vi "Read Unique Employees.vi"(8 "Error In":errorcluster, 11 "DVR In":refnum<data-value>) -> (0 "Error Out":errorcluster, 2 "Unique Employees":string[][](array[string]), 3 "DVR Out":refnum<data-value>)   [LabVIEW 2017, in "Data Operations.lvlib"]
uses:
  Data Operations.lvlib
  Private Controls/Report Data Cluster.ctl
  Private Controls/Data Raw.ctl
panel:
  out "Data":T1[](array[typedef])
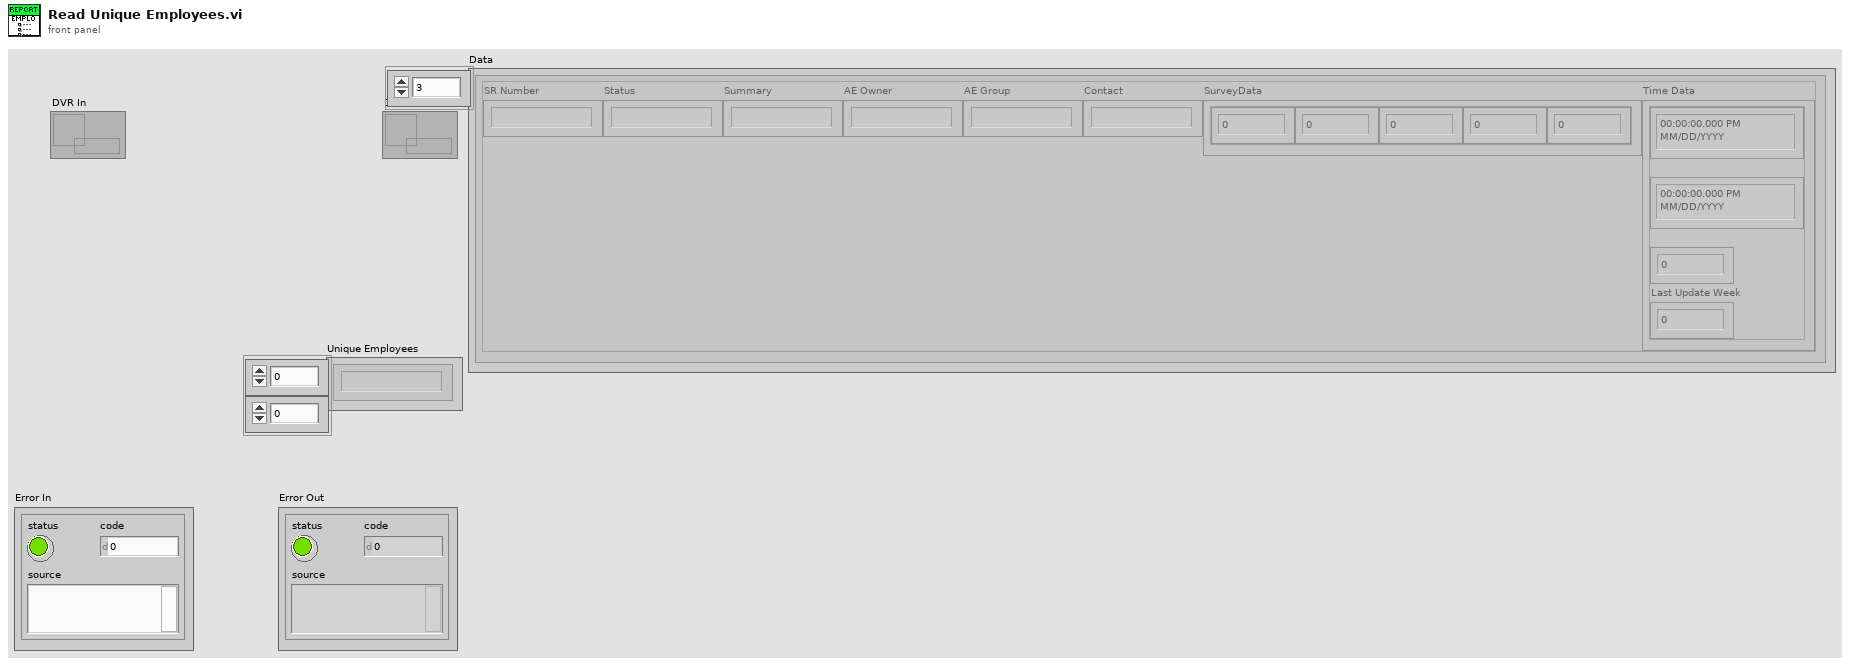
[diagram p1: front panel]
types:
  T1 = typedef "Data Operations.lvlib/Data Raw.ctl" = cluster{"SR Number":string, "Status":string, "Summary":string, "AE Owner":string, "AE Group":string, "Contact":string, "SurveyData":cluster{"Resolution Time":dbl, "Total Satisfaction":dbl, "Response Time":dbl, "Courtesy":dbl, "Problem Solved":dbl}, "Time Data":cluster{"Last Update Date":timestamp, "Creation Date":timestamp, "Creation week":u8, "Last Update Week":u8}}
  T2 = typedef "Data Operations.lvlib/Report Data Cluster.ctl" = cluster{"Headers":cluster{"Start Date":timestamp, "End Date":timestamp, "SR Status String":string[], "AE Owner String":string[]}, "Data":T1[]}
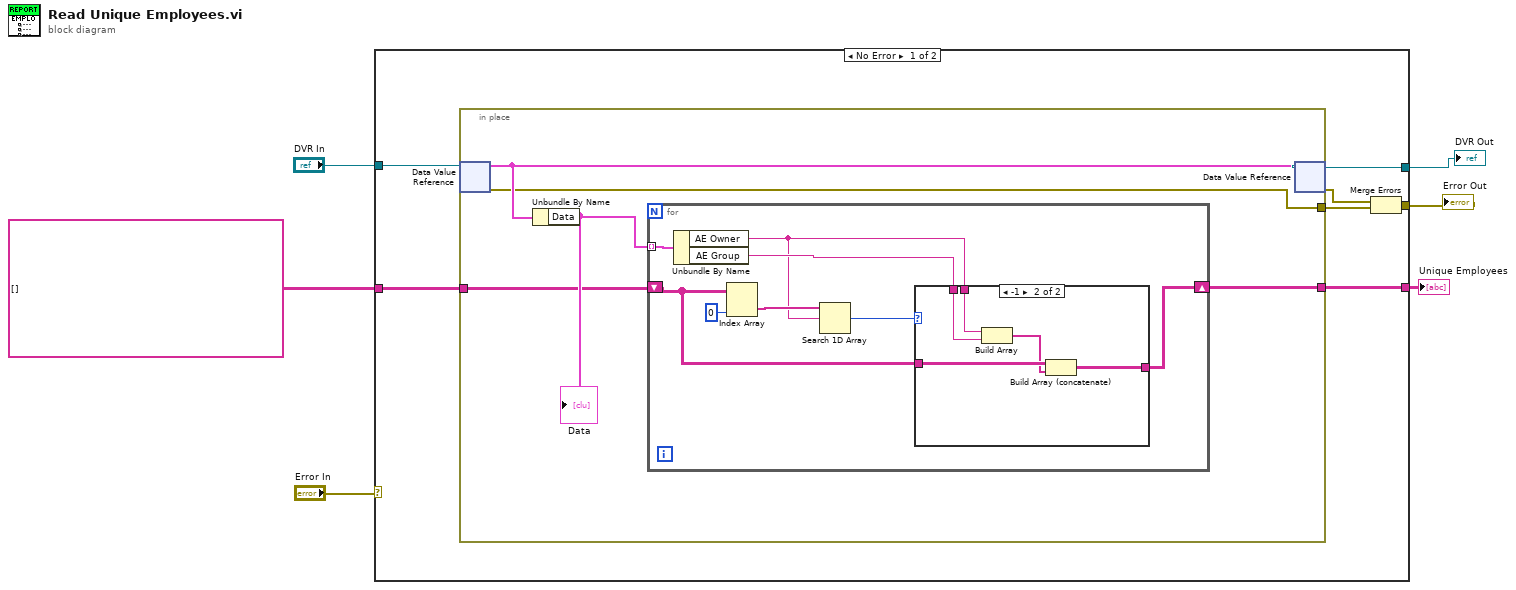
[diagram p0: block diagram]
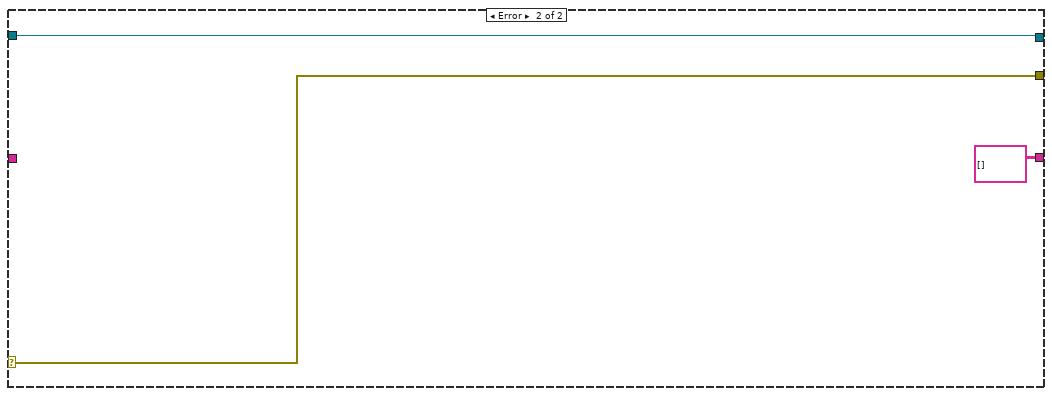
[diagram p3: hidden frame]
diagram:
  n1 = case shown="No Error" "Error In" {
    selector: "Error In" -> [_ w35]
    tunnel: "DVR In" -> [w13 w34]
    tunnel: [w10 w35] -> w5
    tunnel: [w9 w34] -> w3
    tunnel: string[][] [] -> [w8 _]
    tunnel: [w7 string[][] []] -> w1
    frame No Error {
      n2 = in-place {
        in-place-border: [w17] -> w11
        in-place-border: w8 -> [w15]
        in-place-border: [w14] -> w7
        n3 = in-place-dvr #1(w13) -> (w18:T2, w17:errorcluster)
        n4 = Unbundle By Name(w18) -> ("Data"=w16:T1[])
        "Data" <- w16
        n5 = for {
          tunnel: w16 -> [w26] mode=indexing
          shift-right: [w20] -> w14
          shift-left: w15 -> [w22]
          n6 = Unbundle By Name(w26) -> ("AE Owner"=w19:string, "AE Group"=w21:string)
          n7 = Index Array(array=w22, index (col)=0 ("disabled index (col)")) -> (element=w24:string[])  [unwired: 1 in]
          n8 = Search 1D Array(1D array=w24, element=w19) -> (index of element=w23:i32)  [unwired: 1 in]
          n9 = case shown="-1" w23 {
            tunnel: w22 -> [w27 w32]
            tunnel: w19 -> [_ w31]
            tunnel: w21 -> [_ w30]
            tunnel: [w27 w28] -> w20
            frame Default {
            }
            frame -1 {
              n10 = Build Array(w31, w30) -> (w29:string[])
              n11 = Build Array (concatenate)(w32, w29) -> (w28:string[][])
            }
          }
        }
        n12 = in-place-dvr #1(w18) -> (w9:refnum<data-value>, w12:errorcluster)
      }
      n13 = Merge Errors(w12, w11) -> (w10:errorcluster)
    }
    frame Error {
    }
  }
  "Error Out" <- w5
  "DVR Out" <- w3
  "Unique Employees" <- w1
